vi "removeChild.vi"(0 "reference":refnum<class "AbstractNode.lvclass">, 1 "node":refnum<class "AbstractNode.lvclass">, 5 "error in (no error)":errorcluster) -> (14 "reference out":refnum<class "AbstractNode.lvclass">, 19 "error out":errorcluster)   [LabVIEW 2012, in "AbstractNode.lvclass"]
doc: "public void removeChild(Node node)"
uses:
  <resource>/Framework/Providers/Open_GDS/UML/AbstractNode_class/AbstractNode.lvclass
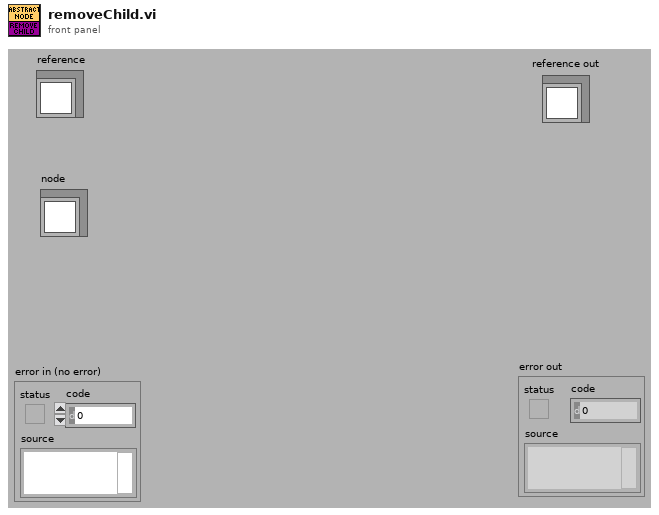
[diagram p1: front panel]
types:
  T1 = typedef "AbstractNode.lvclass/ObjectAttributes.ctl" = cluster{"parent":refnum<class "AbstractNode.lvclass">, "children":refnum<class "AbstractNode.lvclass">[], "Hidden":bool}
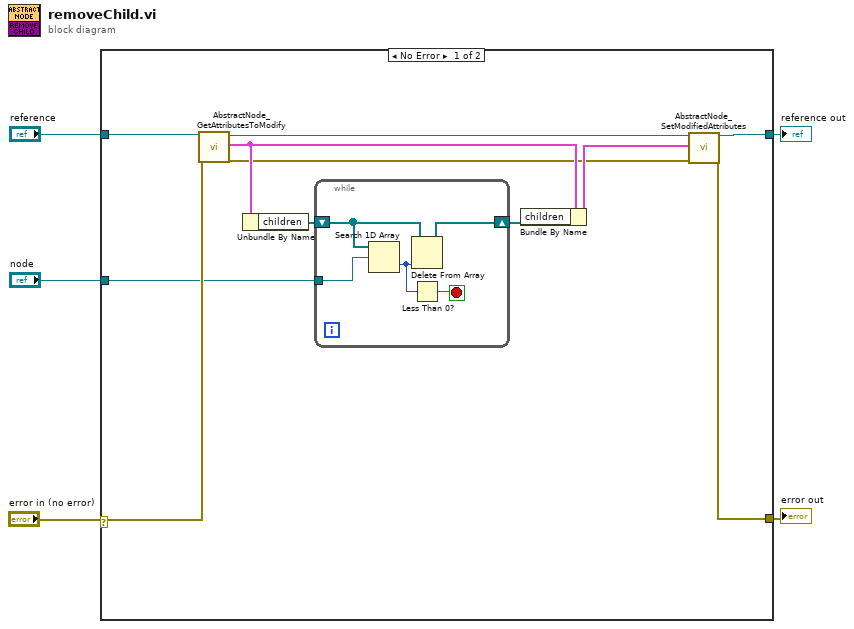
[diagram p0: block diagram]
diagram:
  n1 = case shown="No Error" "error in (no error)" {
    selector: "error in (no error)" -> [w13 w22]
    tunnel: "reference" -> [w16 w23]
    tunnel: [w15 w22] -> w4
    tunnel: [w14 w23] -> w3
    tunnel: "node" -> [w12 _]
    frame No Error {
      n2 = call <resource>:"AbstractNode_GetAttributesToModify.vi"("reference in"=w16, "error in (no error)"=w13) -> ("reference out"=w11:refnum<class "AbstractNode.lvclass">, "Attributes"=w10:T1, "error out"=w6:errorcluster)  [unwired: 1 in, 14 out]
      n3 = Unbundle By Name(w10) -> ("children"=w7:refnum<class "AbstractNode.lvclass">[])
      n4 = while {
        tunnel: w12 -> [w21]
        shift-right: [w20] -> w8
        shift-left: w7 -> [w19]
        stop <- w17 stop-if-true
        n5 = Search 1D Array(1D array=w19, element=w21) -> (index of element=w18:i32)  [unwired: 1 out]
        n6 = Delete From Array(array=w19, index=w18) -> (array with subset deleted=w20:refnum<class "AbstractNode.lvclass">[])  [unwired: 1 in, 1 out]
        n7 = Less Than 0?(x=w18) -> (x < 0?=w17:bool)
      }
      n8 = Bundle By Name(cluster=w10, "children"=w8) -> (w9:T1)
      n9 = call <resource>:"AbstractNode_SetModifiedAttributes.vi"("reference in"=w11, "Attributes"=w9, "error in (no error)"=w6) -> ("reference out"=w14:refnum<class "AbstractNode.lvclass">, "error out"=w15:errorcluster)  [unwired: 3 in, 12 out]
    }
    frame Error {
    }
  }
  "reference out" <- w3
  "error out" <- w4
